vi "Enqueue Task List.vi"(8 "error in (no error)":errorcluster, 11 "BuildWorker in":refnum<class "BuildWorker.lvclass">) -> (0 "error out":errorcluster, 3 "BuildWorker out":refnum<class "BuildWorker.lvclass">)   [LabVIEW 2017, in "BuildWorker.lvlib" / "BuildWorker.lvclass"]
uses:
  BuildWorker.lvclass
  BuildWorker.lvclass/BuildWorker.ctl
  Classes/Task Interface/Task/Status.ctl
  Classes/Task Interface/Task/Task.lvclass/Task.ctl
  Classes/Task Interface/Task/Get Name.vi
  Classes/Task Interface/Task/Task.lvclass
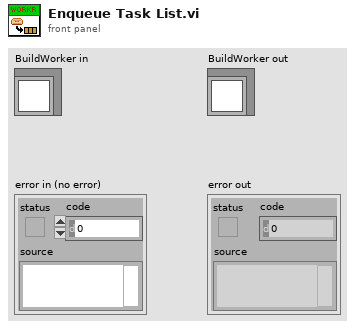
[diagram p1: front panel]
types:
  T1 = typedef "Task Interface.lvlib/Task.lvclass/Status.ctl" = enum16{"Created", "Added", "Pending", "Queued", "Processing", "Cleaning", "Building", "Finished", "Failed", "Removed", "Not found"}
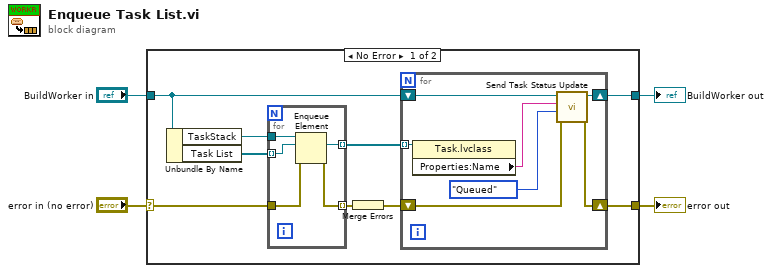
[diagram p0: block diagram]
diagram:
  n1 = case shown="No Error" "error in (no error)" {
    selector: "error in (no error)" -> [w11 w26]
    tunnel: [w7 w26] -> w3
    tunnel: [w6 w25] -> w1
    tunnel: "BuildWorker in" -> [w9 w25]
    frame No Error {
      n2 = Unbundle By Name(w9) -> ("TaskStack"=w13:refnum<queue>, "Task List"=w12:refnum<class "Task.lvclass">[])
      n3 = for {
        tunnel: w13 -> [w24]
        tunnel: w12 -> [w21] mode=indexing
        tunnel: w11 -> [w23]
        tunnel: [w22] -> w10 mode=indexing
        tunnel: [w21] -> w5 mode=indexing
        n4 = Enqueue Element(queue=w24, element=w21, error in (no error)=w23) -> (error out=w22:errorcluster)  [unwired: 1 in, 2 out]
      }
      n5 = Merge Errors(w10) -> (w8:errorcluster)
      n6 = for {
        shift-right: [w19] -> w6
        shift-left: w9 -> [w20]
        shift-right: [w17] -> w7
        shift-left: w8 -> [w18]
        tunnel: w5 -> [w16] mode=indexing
        n7 = property class="Task.lvclass"(reference=w16) -> ("Properties:Name"=w15:string)  [unwired: 1 in, 2 out]
        n8 = call "Send Task Status Update.vi"("error in (no error)"=w18, "Status"=Status."Queued", "Task Name"=w15, "BuildWorker in"=w20) -> ("error out"=w17:errorcluster, "BuildWorker out"=w19:refnum<class "BuildWorker.lvclass">)  [unwired: 6 in]
      }
    }
    frame Error {
    }
  }
  "error out" <- w3
  "BuildWorker out" <- w1
